vi "SaveWWWImages.vi"(7 "Tab charts":refnum<vi>, 9 "Main":refnum<vi>, 10 "Destination":path, 11 "VI in":refnum<vi>) -> ()   [LabVIEW 2017]
panel:
  out "Write Imegtime":u32
  out "get Imegtime":u32
  out "Time":u32
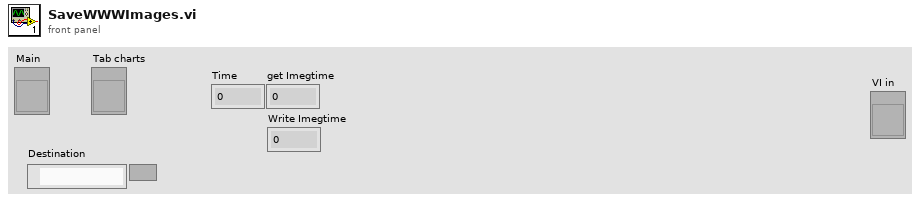
[diagram p1: front panel]
types:
  T1 = typedef "imagedata.ctl" = cluster{"image type":i32, "image depth":i32, "image":u8[], "mask":u8[], "colors":u32[], "Rectangle":cluster{"left":i16, "top":i16, "right":i16, "bottom":i16}}
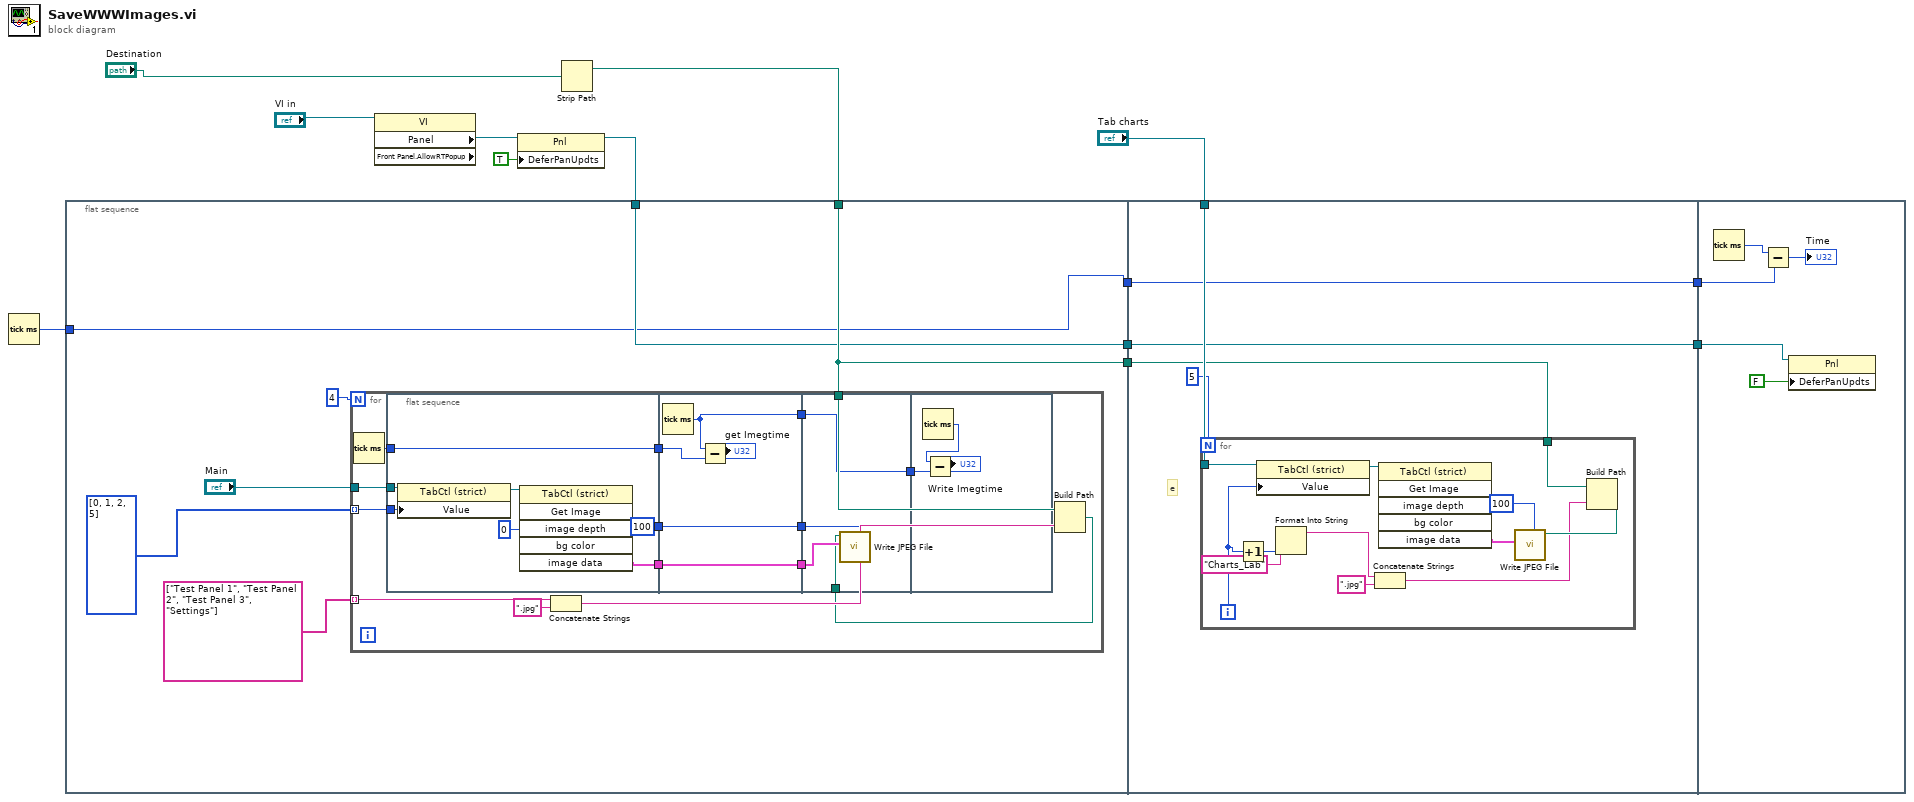
[diagram p0: block diagram]
diagram:
  n1 = Tick Count (ms)() -> (millisecond timer value=w2:u32)
  n2 = flat-sequence {
    tunnel: w9 -> [w17]
    tunnel: w8 -> [w16]
    tunnel: [w17] -> w6
    tunnel: [w16] -> w4
    tunnel: [w15] -> w3
    tunnel: w2 -> [w15]
    tunnel: "Tab charts" -> [w59]
    tunnel: w6 -> [w57]
    tunnel: [w56] -> w5
    tunnel: w4 -> [w56]
    tunnel: w3 -> [w55]
    tunnel: [w55] -> w1
    tunnel: w5 -> [w76]
    tunnel: w1 -> [w73]
    frame #0 {
      n3 = for {
        N: 4 -> [_]
        tunnel: "Main" -> [w35]
        tunnel: i32[] [0, 1, 2, 5] -> [w34] mode=indexing
        tunnel: w17 -> [w33]
        tunnel: string[] ["Test Panel 1", "Test Panel 2", "Test Panel 3", "Settings"] -> [w32] mode=indexing
        n4 = Tick Count (ms)() -> (millisecond timer value=w24:u32)
        n5 = flat-sequence {
          tunnel: w35 -> [w42]
          tunnel: w34 -> [w40]
          tunnel: [w39] -> w29
          tunnel: [100 ("quality (80)")] -> w27
          tunnel: [w37] -> w25
          tunnel: w24 -> [w37]
          tunnel: w29 -> [w47]
          tunnel: [w47] -> w28
          tunnel: w27 -> [w46]
          tunnel: [w46] -> w26
          tunnel: w25 -> [w45]
          tunnel: [w43] -> w22
          tunnel: w28 -> [w50]
          tunnel: w26 -> [w51]
          tunnel: w23 -> [w49]
          tunnel: w22 -> [w48]
          tunnel: [w48] -> w21
          tunnel: w21 -> [w52]
          frame #0 {
            n6 = property class="TabCtl (strict)"(reference=w42, "Value"=w40) -> (reference out=w41:refnum<vi>)  [unwired: 1 in, 1 out]
            n7 = invoke class="TabCtl (strict)" method="Get Image"(reference=w41, "image depth"=0 ("Image Depth")) -> ("image data"=w39:T1)  [unwired: 4 in, 5 out]
          }
          frame #1 {
            n8 = Tick Count (ms)() -> (millisecond timer value=w43:u32)
            n9 = Subtract(x=w43, y=w45) -> (x-y=→"get Imegtime":u32)
          }
          frame #2 {
            n10 = call <vilib>:"Write JPEG File.vi"("quality (80)"=w51, "image data"=w50, "path to JPEG file"=w49) -> ()  [unwired: 7 in, 2 out]
          }
          frame #3 {
            n11 = Tick Count (ms)() -> (millisecond timer value=w53:u32)
            n12 = Subtract(x=w53, y=w52) -> (x-y=→"Write Imegtime":u32)
          }
        }
        n13 = Concatenate Strings(w32, ".jpg" ("string")) -> (w30:string)
        n14 = Build Path(base path=w33, name or relative path=w30) -> (appended path=w23:path)
      }
    }
    frame #1 {
      # "e"
      n15 = for {
        N: 5 -> [_]
        tunnel: w59 -> [w71]
        tunnel: w57 -> [w68]
        i -> [w63]
        n16 = Increment(x=w63) -> (x+1=w64:i32)
        n17 = property class="TabCtl (strict)"(reference=w71, "Value"=w63) -> (reference out=w70:refnum<vi>)  [unwired: 1 in, 1 out]
        n18 = Format Into String(initial string="Charts_Lab", w64) -> (resulting string=w61:string)  [unwired: 2 in, 1 out]
        n19 = Concatenate Strings(w61, ".jpg" ("string")) -> (w65:string)
        n20 = invoke class="TabCtl (strict)" method="Get Image"(reference=w70) -> ("image data"=w67:T1)  [unwired: 5 in, 5 out]
        n21 = Build Path(base path=w68, name or relative path=w65) -> (appended path=w69:path)
        n22 = call <vilib>:"Write JPEG File.vi"("quality (80)"=100, "image data"=w67, "path to JPEG file"=w69) -> ()  [unwired: 7 in, 2 out]
      }
    }
    frame #2 {
      n23 = Tick Count (ms)() -> (millisecond timer value=w74:u32)
      n24 = Subtract(x=w74, y=w73) -> (x-y=→"Time":u32)
      n25 = property class="Pnl"(reference=w76, "DeferPanUpdts"=FALSE ("Defer Panel Updates")) -> ()  [unwired: 1 in, 2 out]
    }
  }
  n26 = property class="VI" props=["Panel", "Front Panel.AllowRTPopup"](reference="VI in") -> ("Panel"=w12:refnum<vi>)  [unwired: 1 in, 3 out]
  n27 = property class="Pnl"(reference=w12, "DeferPanUpdts"=TRUE ("Defer Panel Updates")) -> (reference out=w8:refnum<vi>)  [unwired: 1 in, 1 out]
  n28 = Strip Path(path="Destination") -> (stripped path=w9:path)  [unwired: 1 out]
